vi "Test 5 compare Adjacent symbol.vi"(8 "error in (no error)":errorcluster, 11 "Test Case In":refnum<class "Schema parsing test.lvclass">) -> (0 "error out":errorcluster, 3 "Test Case Out":refnum<class "Schema parsing test.lvclass">)   [LabVIEW 2020, in "Schema parsing test.lvclass"]
uses:
  Schema parsing test.lvclass
  C:/Program Files (x86)/National Instruments/LabVIEW 2020/vi.lib/Astemes/LUnit/Test Case.lvclass
  <vilib>/Astemes/LUnit/Test Case.lvclass/Test Case.ctl
  <vilib>/Astemes/LUnit/Append Fail Result.vi
  <vilib>/Astemes/LUnit/Append Pass Result.vi
  Symbol/Symbol.lvclass
  Number/Number.lvclass
  Schema Parser/Schema Parser.lvclass
  <vilib>/Astemes/LUnit/Test Case.lvclass
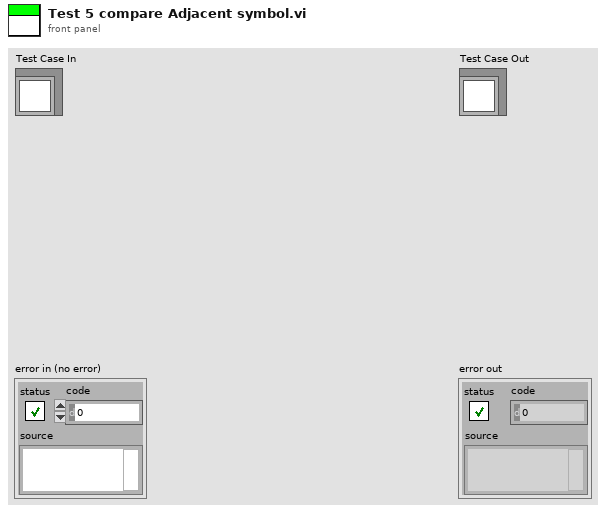
[diagram p1: front panel]
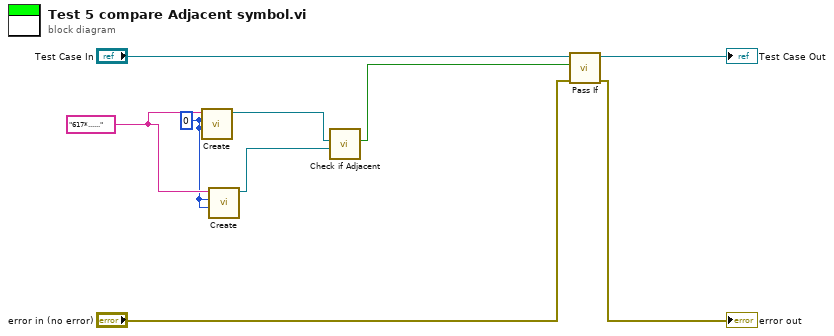
[diagram p0: block diagram]
diagram:
  w4 = 0 ("Col Offset")
  w5 = "617*......" ("String")
  n1 = call "Create.vi"("Row"=w4, "Col Offset"=w4, "String"=w5) -> ("Number"=w3:refnum<class "Number.lvclass">)  [unwired: 6 in, 2 out]
  n2 = call "Create.vi"("Row"=w4, "Col Offset"=w4, "String"=w5) -> ("Number"=w2:refnum<class "Symbol.lvclass">)  [unwired: 6 in, 2 out]
  n3 = call "Check if Adjacent.vi"("Symbol.lvclass"=w2, "Number.lvclass"=w3) -> ("Is Adjacent?"=w1:bool)  [unwired: 8 in, 1 out]
  n4 = call <vilib>:"Pass If.vi"("error in (no error)"="error in (no error)", "Pass?"=w1, "LUnit Test Case In"="Test Case In") -> ("error out"=→"error out":errorcluster, "LUnit Test Case Out"=→"Test Case Out":refnum<class "Schema parsing test.lvclass">)  [unwired: 7 in]
